vi "two-char-cksum.vi"(10 "B":string, 11 "A":string) -> (2 "CKSUM":u8, 3 "concatenated string":string)   [LabVIEW 2014]
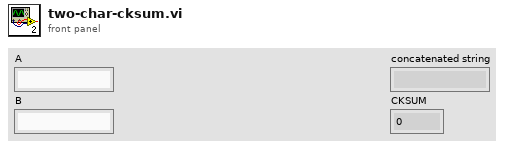
[diagram p1: front panel]
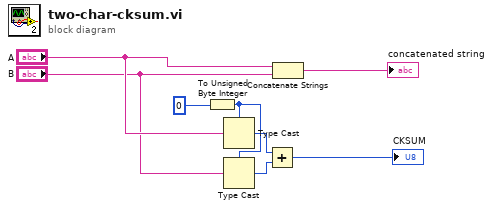
[diagram p0: block diagram]
diagram:
  n1 = To Unsigned Byte Integer(number=0) -> (unsigned 8bit integer=w6:u8)
  n2 = Type Cast(type=w6, x="A") -> (*(type *) &x=w7:u8)
  n3 = Type Cast(type=w6, x="B") -> (*(type *) &x=w5:u8)
  n4 = Add(x=w7, y=w5) -> (x+y=→"CKSUM":u8)
  n5 = Concatenate Strings("A", "B") -> (→"concatenated string":string)
